vi "WSVCAP SHL Host LL I2C Write.vi"(0 "C1 Data Out [DUT Ordered]":u8[][](array[numeric]) format="%.0x", 1 "Wait Ticks":u32, 2 "Slave Address":u8, 5 "C2 Data Out [DUT Ordered]":u8[][](array[numeric]) format="%.0x", 7 "C3 Data Out [DUT Ordered]":u8[][](array[numeric]) format="%.0x", 9 "Socket Mask [U64]":u64=1 format="%016x", 11 "error in":errorcluster, 12 "Sub Address":u8=20) -> (10 "Status":u8[](array[numeric]), 15 "error out":errorcluster)   [LabVIEW 2012]
uses:
  Type Defs/WSVCAP SHL Top Level Write Read State Enum.ctl
  Type Defs/WSVCAP SHL Transaction Enum.ctl
  Type Defs/WSVCAP SHL Top Level Control Enum.ctl
  Type Defs/WSVCAP SHL State.ctl
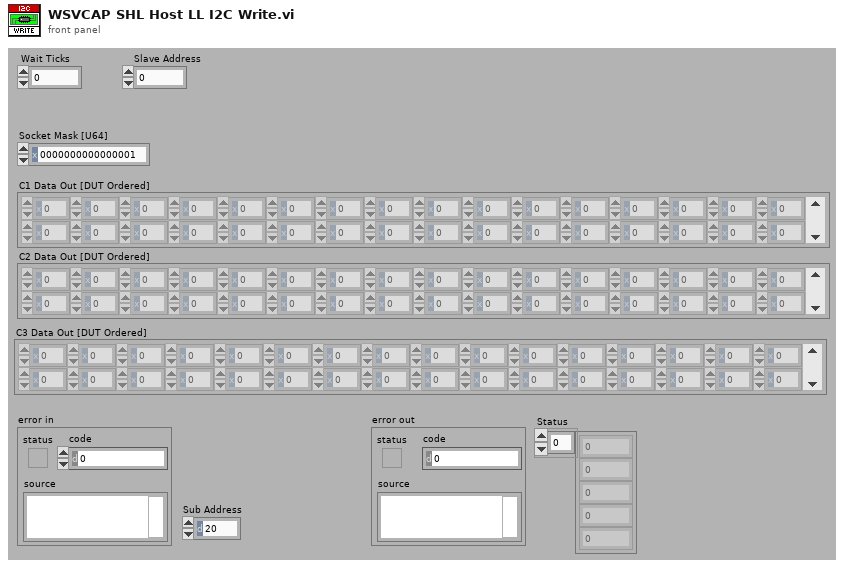
[diagram p1: front panel]
types:
  T1 = typedef "WSVCAP SHL Top Level Write Read State Enum.ctl" = enum16{"Start", "Write", "Read", "Get Status", "Wait Until Done"}
  T2 = typedef "WSVCAP SHL Top Level Control Enum.ctl" = enum16{"Start", "Cmd", "Transaction", "Wait Ticks", "Socket Mask", "Slave Address", "Sub Address", "Bytes to Write", "Bytes to Read", "Write Data", "Write Flag", "Read Data", "Read Flag", "Ack Read", "Read Status Flag", "Ack Read Status", "Status", "Cycle Count", "Stop Cycle", "Exit"}
  T3 = typedef "WSVCAP SHL Transaction Enum.ctl" = enum16{"I2C-Read Data", "I2C-Write Data", "SPI-Write/Read Data", "RFFE-Ext Write", "RFFE-Ext Read"}
  T4 = typedef "WSVCAP SHL State.ctl" = enum8{"Idle", "Transfer Data"}
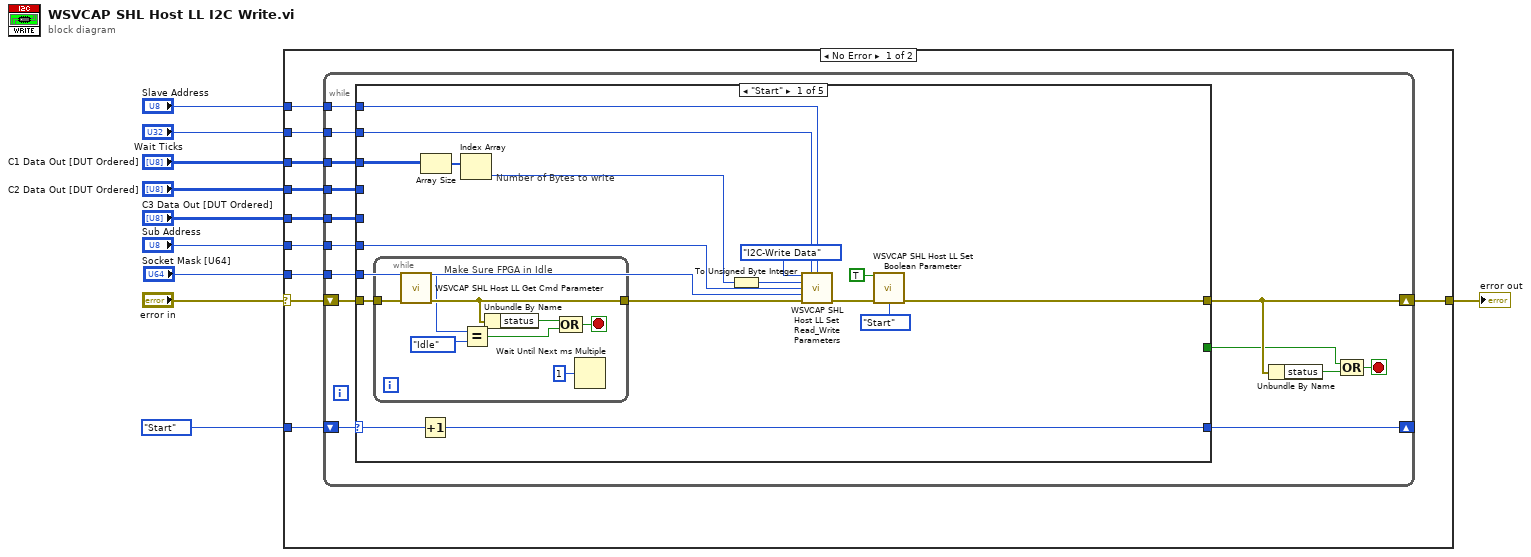
[diagram p0: block diagram]
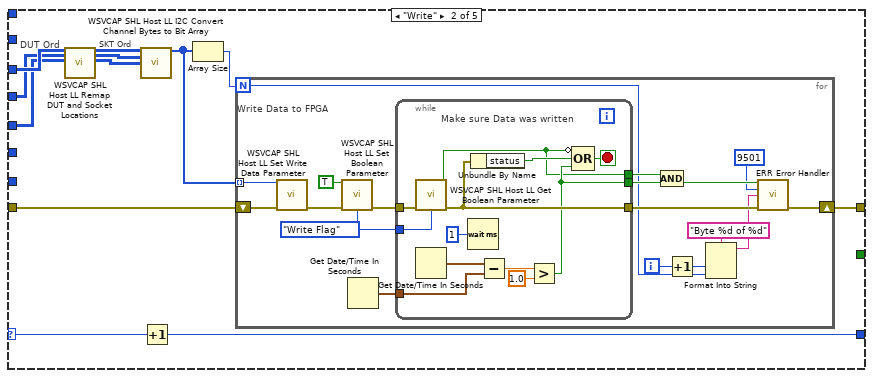
[diagram p2: hidden frame]
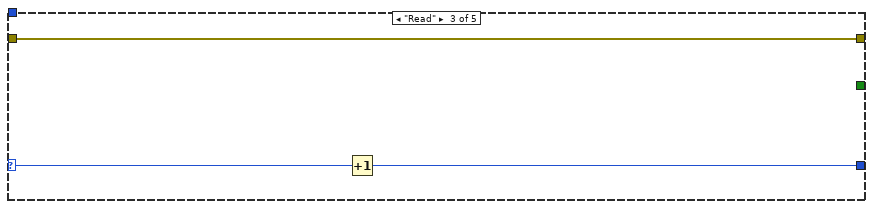
[diagram p3: hidden frame]
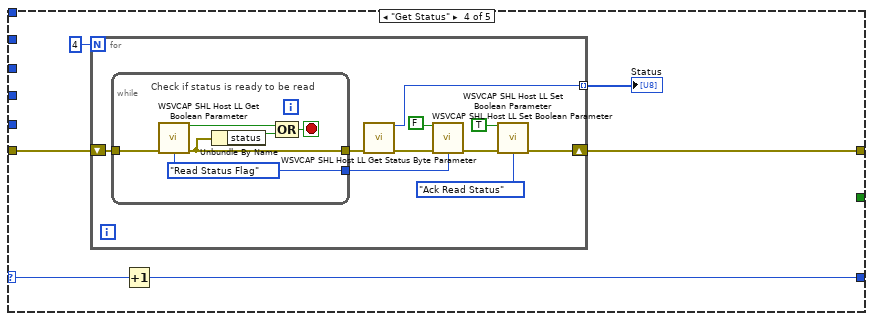
[diagram p4: hidden frame]
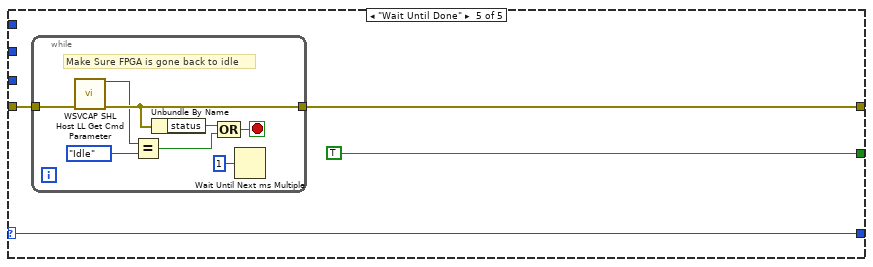
[diagram p5: hidden frame]
diagram:
  n1 = case shown="No Error" "error in" {
    selector: "error in" -> [w14 w138]
    tunnel: [w20 w138] -> w10
    tunnel: WSVCAP_SHL_Top_Level_Write_Read_State_Enum."Start" ("Write Read State") -> [w19 _]
    tunnel: "C1 Data Out [DUT Ordered]" -> [w18 _]
    tunnel: "C2 Data Out [DUT Ordered]" -> [w17 _]
    tunnel: "Sub Address" -> [w16 _]
    tunnel: "Socket Mask [U64]" -> [w15 _]
    tunnel: "Wait Ticks" -> [w13 _]
    tunnel: "C3 Data Out [DUT Ordered]" -> [w12 _]
    tunnel: "Slave Address" -> [w11 _]
    frame No Error {
      n2 = while {
        shift-right: [w33] -> w20
        shift-left: w14 -> [w34]
        shift-right: [w28] -> _
        shift-left: w19 -> [w29]
        tunnel: w18 -> [w27]
        tunnel: w17 -> [w26]
        tunnel: w16 -> [w25]
        tunnel: w15 -> [w24]
        tunnel: w13 -> [w23]
        tunnel: w12 -> [w22]
        tunnel: w11 -> [w21]
        stop <- w30 stop-if-true
        n3 = case shown="\"Start\"" w29 {
          selector: w29 -> [w49 w68 w102 w107 w127]
          tunnel: w34 -> [w50 w61 w103 w109 w129]
          tunnel: [w46 w70 w103 w108 w128] -> w33
          tunnel: [_ _ _ _ TRUE] -> w32
          tunnel: [w48 w69 w101 w106 w127] -> w28
          tunnel: w27 -> [w42 w65 _ _ _]
          tunnel: w26 -> [_ w64 _ _ _]
          tunnel: w25 -> [w38 _ _ _ _]
          tunnel: w24 -> [w37 _ _ _ _]
          tunnel: w23 -> [w36 _ _ _ _]
          tunnel: w22 -> [_ w60 _ _ _]
          tunnel: w21 -> [w35 _ _ _ _]
          frame "Start" {
            # "Number of Bytes to write"
            n4 = while {
              tunnel: w50 -> [w54]
              tunnel: [w53] -> w47
              stop <- w58 stop-if-true
              # "Make Sure FPGA in Idle"
              n5 = call "WSVCAP SHL Host LL Get Cmd Parameter.vi"("error in (no error)"=w54) -> ("I2C_Cmd"=w52:T4, "error out"=w53:errorcluster)  [unwired: 13 in]
              n6 = Equal?(x=w52, y=WSVCAP_SHL_State."Idle" ("Type")) -> (x = y?=w56:bool)
              n7 = Unbundle By Name(w53) -> ("status"=w51:bool)
              n8 = Compound Arithmetic op=OR(w51, w56) -> (w58:bool)
              n9 = Wait Until Next ms Multiple(millisecond multiple=u32 1) -> ()  [unwired: 1 out]
            }
            n10 = Increment(x=w49) -> (x+1=w48:T1)
            n11 = Array Size(array=w42) -> (size(s)=w41:i32[])
            n12 = Index Array(array=w41) -> (element=w40:i32)  [unwired: 1 in]
            n13 = To Unsigned Byte Integer(number=w40) -> (unsigned 8bit integer=w39:u8)
            n14 = call "WSVCAP SHL Host LL Set Read_Write Parameters.vi"("Transaction"=WSVCAP_SHL_Transaction_Enum."I2C-Write Data", "Wait Ticks"=w36, "Slave Address"=w35, "Bytes"=w39, "Sub Address [U8]"=w38, "Socket Mask [U64]"=w37, "error in (no error)"=w47) -> ("error out"=w46:errorcluster)  [unwired: 8 in]
            n15 = call "WSVCAP SHL Host LL Set Boolean Parameter.vi"("Boolean In"=TRUE, "error in (no error)"=w46, "FPGA Top Level Control"=WSVCAP_SHL_Top_Level_Control_Enum."Start") -> ()  [unwired: 12 in, 1 out]
          }
          frame "Write" {
            # "SKT Ord"
            # "DUT Ord"
            # "Write Data to FPGA"
            n16 = call "WSVCAP SHL Host LL Remap DUT and Socket Locations.vi"("C1 DUT Ordered Data In"=w65, "C2 DUT Ordered Data In"=w64, "C3 DUT Ordered Data In"=w60) -> ("C1 Socket Ordered Data Out"=w63:u8[][], "C2 Socket Ordered Data Out"=w62:u8[][], "C3 Socket Ordered Data Out"=w59:u8[][])  [unwired: 11 in, 3 out]
            n17 = call "WSVCAP SHL Host LL I2C Convert Channel Bytes to Bit Array.vi"("C1 Data Out"=w63, "C2 Data Out"=w62, "C3 Data Out"=w59) -> ("Write Data"=w66:u64[])  [unwired: 12 in]
            n18 = Increment(x=w68) -> (x+1=w69:T1)
            n19 = Array Size(array=w66) -> (size(s)=w67:i32)
            n20 = for {
              N: w67 -> [w72]
              shift-right: [w80] -> w70
              shift-left: w61 -> [w88]
              tunnel: w66 -> [w87] mode=indexing
              i -> [w75]
              w83 = WSVCAP_SHL_Top_Level_Control_Enum."Write Flag" ("FPGA Top Level Control")
              n21 = call "WSVCAP SHL Host LL Set Write Data Parameter.vi"("Write Byte In"=w87, "error in (no error)"=w88) -> ("error out"=w86:errorcluster)  [unwired: 13 in]
              n22 = call "WSVCAP SHL Host LL Set Boolean Parameter.vi"("Boolean In"=TRUE, "error in (no error)"=w86, "FPGA Top Level Control"=w83) -> ("error out"=w84:errorcluster)  [unwired: 12 in]
              n23 = Get Date/Time In Seconds() -> (seconds since 1Jan1904=w82:timestamp)
              n24 = while {
                tunnel: w84 -> [w98]
                tunnel: [w97] -> w81
                tunnel: w83 -> [w96]
                tunnel: w82 -> [w93]
                tunnel: [w90] -> w79
                tunnel: [w89] -> w78
                stop <- w100 stop-if-true
                # "Make sure Data was written"
                n25 = call "WSVCAP SHL Host LL Get Boolean Parameter.vi"("error in (no error)"=w98, "FPGA Top Level Control"=w96) -> ("Boolean Out"=w89:bool, "error out"=w97:errorcluster)  [unwired: 12 in]
                n26 = Get Date/Time In Seconds() -> (seconds since 1Jan1904=w94:timestamp)
                n27 = Wait (ms)(milliseconds to wait=u32 1) -> ()  [unwired: 1 out]
                n28 = Unbundle By Name(w97) -> ("status"=w95:bool)
                n29 = Subtract(x=w94, y=w93) -> (x-y=w92:dbl)
                n30 = Greater?(x=w92, y=1.0) -> (0:w90:bool)
                n31 = Compound Arithmetic op=OR(invert w89, w95, w90) -> (w100:bool)
              }
              n32 = Compound Arithmetic op=AND(w78, w79) -> (w77:bool)
              n33 = Increment(x=w75) -> (x+1=w71:i32)
              n34 = Format Into String(format string="Byte %d of %d", w71, w72) -> (resulting string=w74:string)  [unwired: 2 in, 1 out]
              n35 = call "ERR Error Handler.vi"("Error Status"=w77, "Error Code"=9501, "Cause Of Error"=w74, "Error In (no error)"=w81) -> ("Error Out"=w80:errorcluster)  [unwired: 11 in]
            }
          }
          frame "Read" {
            n36 = Increment(x=w102) -> (x+1=w101:T1)
          }
          frame "Get Status" {
            n37 = for {
              N: 4 -> [_]
              shift-right: [w118] -> w108
              shift-left: w109 -> [w119]
              tunnel: [w110] -> w104 mode=indexing
              n38 = while {
                tunnel: w119 -> [w123]
                tunnel: [w122] -> w117
                tunnel: [w120] -> w115
                stop <- w125 stop-if-true
                w120 = WSVCAP_SHL_Top_Level_Control_Enum."Read Status Flag" ("FPGA Top Level Control")
                # "Check if status is ready to be read"
                n39 = call "WSVCAP SHL Host LL Get Boolean Parameter.vi"("error in (no error)"=w123, "FPGA Top Level Control"=w120) -> ("Boolean Out"=w124:bool, "error out"=w122:errorcluster)  [unwired: 12 in]
                n40 = Unbundle By Name(w122) -> ("status"=w121:bool)
                n41 = Compound Arithmetic op=OR(w124, w121) -> (w125:bool)
              }
              n42 = call "WSVCAP SHL Host LL Get Status Byte Parameter.vi"("error in (no error)"=w117) -> ("I2C Status Byte"=w110:u8, "error out"=w116:errorcluster)  [unwired: 13 in]
              n43 = call "WSVCAP SHL Host LL Set Boolean Parameter.vi"("Boolean In"=FALSE ("Read Flag"), "error in (no error)"=w116, "FPGA Top Level Control"=w115) -> ("error out"=w111:errorcluster)  [unwired: 12 in]
              n44 = call "WSVCAP SHL Host LL Set Boolean Parameter.vi"("Boolean In"=TRUE ("Write Flag"), "error in (no error)"=w111, "FPGA Top Level Control"=WSVCAP_SHL_Top_Level_Control_Enum."Ack Read Status") -> ("error out"=w118:errorcluster)  [unwired: 12 in]
            }
            "Status" <- w104
            n45 = Increment(x=w107) -> (x+1=w106:T1)
          }
          frame "Wait Until Done" {
            n46 = while {
              tunnel: w129 -> [w132]
              tunnel: [w131] -> w128
              stop <- w134 stop-if-true
              # "Make Sure FPGA is gone back to idle"
              n47 = call "WSVCAP SHL Host LL Get Cmd Parameter.vi"("error in (no error)"=w132) -> ("I2C_Cmd"=w130:T4, "error out"=w131:errorcluster)  [unwired: 13 in]
              n48 = Equal?(x=w130, y=WSVCAP_SHL_State."Idle") -> (x = y?=w135:bool)
              n49 = Unbundle By Name(w131) -> ("status"=w136:bool)
              n50 = Compound Arithmetic op=OR(w136, w135) -> (w134:bool)
              n51 = Wait Until Next ms Multiple(millisecond multiple=u32 1) -> ()  [unwired: 1 out]
            }
          }
        }
        n52 = Unbundle By Name(w33) -> ("status"=w31:bool)
        n53 = Compound Arithmetic op=OR(w32, w31) -> (w30:bool)
      }
    }
    frame Error {
    }
  }
  "error out" <- w10
